vi "ukol5.vi"() -> ()   [LabVIEW 2023]
uses:
  <vilib>/Utility/file.llb/Read Delimited Spreadsheet (DBL).vi
panel:
  out "XY Graph":cluster{"Array":dbl[], "x/y 2":dbl[]}(graph)
  out "Waveform Graph":waveform(dbl)(graph)
  out "appended path":path
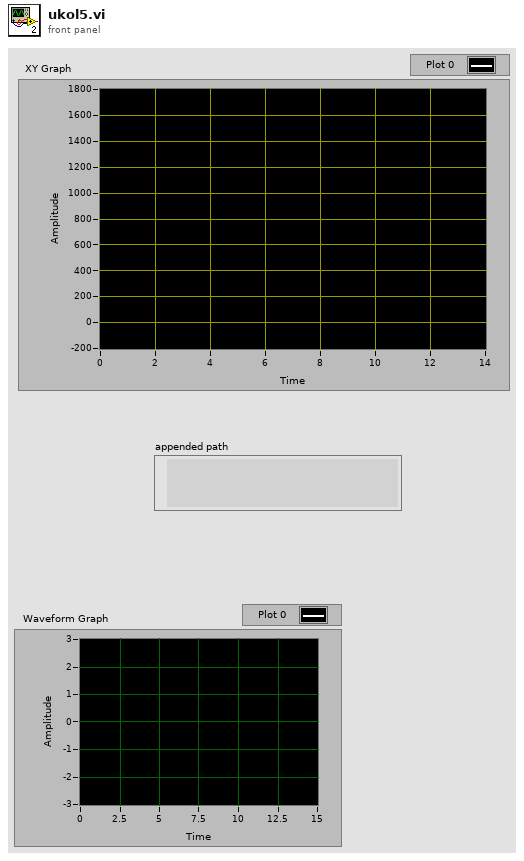
[diagram p1: front panel]
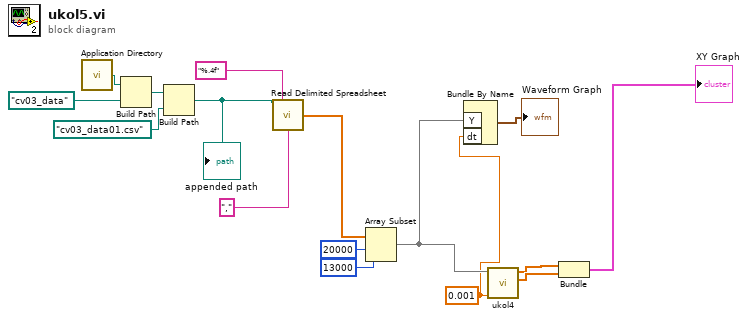
[diagram p0: block diagram]
diagram:
  w2 = 0.001 ("dt")
  n1 = call <vilib>:"Application Directory.vi"() -> ("Application Directory"=w16:path)
  n2 = Build Path(base path=w16, name or relative path=path "cv03_data") -> (appended path=w15:path)
  n3 = Build Path(base path=w15, name or relative path=path "cv03_data01.csv") -> (appended path=w10:path)
  "appended path" <- w10
  n4 = call-poly <vilib>:"Read Delimited Spreadsheet.vi"("file path (dialog if empty)"=w10, "format (%.3f)"="%.4f", "delimiter (\\t)"="," ("delimiter (\\t)")) -> ("first row"=w9:dbl[])  [unwired: 7 in, 5 out]
  n5 = Array Subset(array=w9, index=20000, length=13000) -> (w3:dbl[])
  n6 = Bundle By Name("Y"=w3, "dt"=w2) -> (→"Waveform Graph":waveform(dbl))  [unwired: 1 in]
  n7 = call "ukol4.vi"("dt"=w2, "Y"=w3) -> ("x/y 2"=w6:dbl[], "Array"=w5:dbl[])  [unwired: 6 in, 2 out]
  n8 = Bundle("Array"=w5, "x/y 2"=w6) -> (→"XY Graph":cluster{"Array":dbl[], "x/y 2":dbl[]})  [unwired: 1 in]
